vi "SettingManagerRestore.vi"(7 "Dummy prefix":string="???? ", 8 "error in (no error)":errorcluster, 9 "Tag":string, 10 "Control Tree":refnum<vi>, 11 "Saved Settings":refnum<vi>) -> (0 "error out":errorcluster)   [LabVIEW 2019]
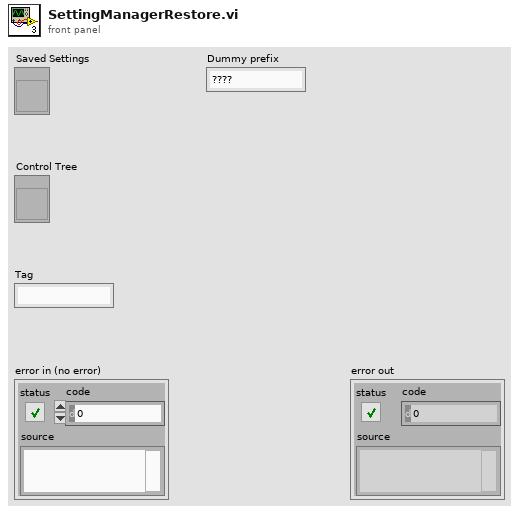
[diagram p1: front panel]
types:
  T1 = typedef "SavedSettingsOptions.ctl" = cluster{"OpenVIs":bool, "RunVIs":bool, "RestoreSubItems":bool, "WaitAfter":u32}
  T2 = enum16{"Left Button", "Center Button", "Right Button", "Window Close"}
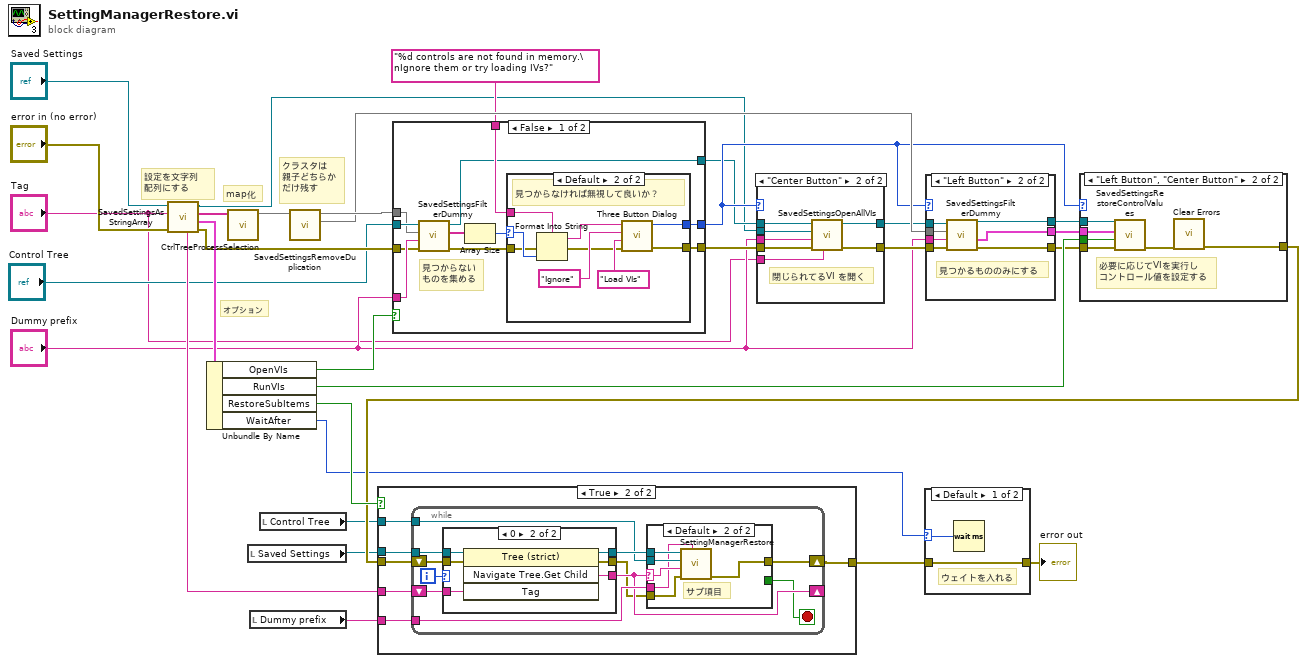
[diagram p0: block diagram]
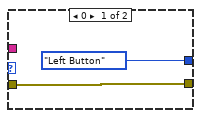
[diagram p2: hidden frame]
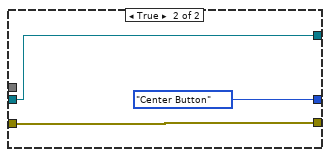
[diagram p3: hidden frame]
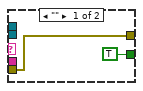
[diagram p9: hidden frame]
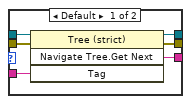
[diagram p10: hidden frame]
diagram:
  # "オプション"
  # "設定を文字列\n配列にする"
  # "クラスタは\n親子どちらか\nだけ残す"
  # "map化"
  n1 = call "SavedSettingsAsStringArray.vi"("error in (no error)"="error in (no error)", "Tag"="Tag", "SavedSettings in"="Saved Settings") -> ("error out"=w18:errorcluster, "Options"=w32:T1, "Selection"=w28:string[], "SavedSettings out"=w7:refnum<vi>, "Active Tag"=w22:string)  [unwired: 4 in]
  n2 = Unbundle By Name(w32) -> ("OpenVIs"=w26:bool, "RunVIs"=w25:bool, "RestoreSubItems"=w24:bool, "WaitAfter"=w21:u32)
  n3 = call "CtrlTreeProcessSelection.vi"("Selection"=w28) -> ("Map"=w29:map{string, string})  [unwired: 10 in]
  n4 = local read "Saved Settings"() -> (w4:refnum<vi>)
  n5 = local read "Dummy prefix"() -> (w5:string)
  n6 = local read "Control Tree"() -> (w3:refnum<vi>)
  n7 = call "SavedSettingsRemoveDuplication.vi"("Saved Values"=w29) -> ("Saved Values (parents removed)"=w27:map{string, string}, "Saved Values (children removed)"=w30:map{string, string})  [unwired: 9 in]
  n8 = case shown="False" w26 {
    tunnel: "Control Tree" -> [w43 w54]
    tunnel: [w42 T2."Center Button" ("Which Button?")] -> w14
    tunnel: w30 -> [w41 _]
    tunnel: "Dummy prefix" -> [w39 _]
    tunnel: w18 -> [w38 w55]
    tunnel: [w36 w55] -> w17
    tunnel: "%d controls are not found in memory.\nIgnore them or try loading IVs?" ("format string") -> [w34 _]
    tunnel: [w33 w54] -> w9
    frame False {
      # "見つからない\nものを集める"
      n9 = call "SavedSettingsFilterDummy.vi"("error in (no error)"=w38, "Dummy prefix"=w39, "Saved Values"=w41, "Control Tree in"=w43) -> ("error out"=w37:errorcluster, "Items Not Found"=w35:string[], "Control Tree out"=w33:refnum<vi>)  [unwired: 4 in, 1 out]
      n10 = Array Size(array=w35) -> (size(s)=w40:i32)
      n11 = case shown="0" w40 {
        selector: w40 -> [_ w53]
        tunnel: [T2."Left Button" ("Which Button?") w49] -> w42
        tunnel: w37 -> [w44 w48]
        tunnel: [w44 w47] -> w36
        tunnel: w34 -> [_ w46]
        frame 0 {
        }
        frame Default {
          # "見つからなければ無視して良いか？"
          n12 = Format Into String(format string=w46, error in=w48, w53) -> (resulting string=w52:string, error out=w47:errorcluster)  [unwired: 1 in]
          n13 = call <vilib>:"Three Button Dialog.vi"("Center Button Text (\"No\")"="Load VIs" ("Center Button Text (\"No\")"), "Left Button Text (\"Yes\")"="Ignore" ("T button name (\"OK\")"), "message"=w52) -> ("Which Button?"=w49:T2)  [unwired: 8 in]
        }
      }
    }
    frame True {
    }
  }
  n14 = case shown="\"Center Button\"" w14 {
    tunnel: w7 -> [_ w65]
    tunnel: w9 -> [w57 w63]
    tunnel: "Dummy prefix" -> [_ w64]
    tunnel: w17 -> [w58 w62]
    tunnel: [w58 w61] -> w16
    tunnel: [w57 w60] -> w12
    tunnel: "Tag" -> [_ w59]
    frame Default {
    }
    frame "Center Button" {
      # "閉じられてるVI を開く"
      n15 = call "SavedSettingsOpenAllVIs.vi"("Tag"=w59, "error in (no error)"=w62, "Dummy prefix"=w64, "Saved Settings"=w65, "Control Tree in"=w63) -> ("error out"=w61:errorcluster, "Control Tree out"=w60:refnum<vi>)  [unwired: 5 in]
    }
  }
  n16 = case shown="\"Left Button\"" w14 {
    tunnel: w27 -> [w69 w76]
    tunnel: [w68 w73] -> w31
    tunnel: "Dummy prefix" -> [_ w75]
    tunnel: w12 -> [w66 w77]
    tunnel: w16 -> [w67 w74]
    tunnel: [w67 w72] -> w15
    tunnel: [w66 w71] -> w11
    frame Default {
      n17 = for {
        tunnel: w69 -> [w70] mode=indexing
        tunnel: [w70] -> w68 mode=indexing
      }
    }
    frame "Left Button" {
      # "見つかるもののみにする"
      n18 = call "SavedSettingsFilterDummy.vi"("error in (no error)"=w74, "Dummy prefix"=w75, "Saved Values"=w76, "Control Tree in"=w77) -> ("error out"=w72:errorcluster, "Items Found"=w73:cluster{string, string}[], "Control Tree out"=w71:refnum<vi>)  [unwired: 4 in, 1 out]
    }
  }
  n19 = case shown="\"Left Button\", \"Center Button\"" w14 {
    tunnel: w11 -> [_ w84]
    tunnel: w31 -> [_ w83]
    tunnel: w25 -> [_ w81]
    tunnel: [w78 w80] -> w23
    tunnel: w15 -> [w78 w79]
    frame Default {
    }
    frame "Left Button", "Center Button" {
      # "必要に応じてVIを実行し\nコントロール値を設定する"
      n20 = call "SavedSettingsRestoreControlValues.vi"("error in (no error)"=w79, "Run VIs"=w81, "SavedValues"=w83, "ControlTree in"=w84) -> ("error out"=w82:errorcluster)  [unwired: 6 in, 1 out]
      n21 = call <vilib>:"Clear Errors.vi"("error in (no error)"=w82) -> ("error out"=w80:errorcluster)  [unwired: 5 in, 1 out]
    }
  }
  n22 = case shown="True" w24 {
    tunnel: w23 -> [w85 w90]
    tunnel: w4 -> [_ w91]
    tunnel: w22 -> [_ w89]
    tunnel: w3 -> [_ w88]
    tunnel: w5 -> [_ w87]
    tunnel: [w85 w86] -> w20
    frame False {
    }
    frame True {
      n23 = while {
        tunnel: w91 -> [w102]
        tunnel: w88 -> [w98]
        tunnel: w87 -> [w97]
        shift-right: [w95] -> _
        shift-left: w89 -> [w100]
        shift-right: [w92] -> w86
        shift-left: w90 -> [w101]
        i -> [w96]
        stop <- w94 stop-if-true
        n24 = case shown="0" w96 {
          tunnel: w102 -> [w116 w122]
          tunnel: w101 -> [w114 w121]
          tunnel: w100 -> [w113 w120]
          tunnel: [w115 w119] -> w99
          tunnel: [w112 w118] -> w95
          tunnel: [w111 w117] -> w93
          frame Default {
            n25 = invoke class="Tree (strict)" method="Navigate Tree.Get Next"(reference=w116, error in=w114, "Tag"=w113) -> (reference out=w115:refnum<vi>, error out=w111:errorcluster, "Navigate Tree:Get Next Item"=w112:string)  [unwired: 1 in, 1 out]
          }
          frame 0 {
            n26 = invoke class="Tree (strict)" method="Navigate Tree.Get Child"(reference=w122, error in=w121, "Tag"=w120) -> (reference out=w119:refnum<vi>, error out=w117:errorcluster, "Navigate Tree:Get Child"=w118:string)  [unwired: 1 in, 1 out]
          }
        }
        n27 = case shown="Default" w95 {
          selector: w95 -> [_ w108]
          tunnel: w99 -> [_ w110]
          tunnel: w98 -> [_ w109]
          tunnel: w97 -> [_ w107]
          tunnel: [TRUE _] -> w94
          tunnel: w93 -> [w103 w106]
          tunnel: [w103 w105] -> w92
          frame "" {
          }
          frame Default {
            # "サブ項目"
            n28 = call "SettingManagerRestore.vi"("Dummy prefix"=w107, "error in (no error)"=w106, "Tag"=w108, "Control Tree"=w109, "Saved Settings"=w110) -> ("error out"=w105:errorcluster)  [unwired: 6 in]
          }
        }
      }
    }
  }
  n29 = case shown="Default" w21 {
    selector: w21 -> [w124 _]
    tunnel: w20 -> [w123 w125]
    tunnel: [w123 w125] -> w2
    frame Default {
      # "ウェイトを入れる"
      n30 = Wait (ms)(milliseconds to wait=w124) -> ()  [unwired: 1 out]
    }
    frame 0 {
    }
  }
  "error out" <- w2
